vi "Graphene Flexion Test.vi"() -> ()   [LabVIEW 2016]
uses:
  <vilib>/rvi/Emulation/niFpgaGetClockAttributes.vi
  <vilib>/rvi/Emulation/niFpgaSctlEmulationGetInTimedLoop.vi
  <vilib>/rvi/Emulation/niFpgaEmulationReportErrorSimple.vi
  <vilib>/rvi/eio/common/nirviEmuTemplateMethod_errors.vi
  <vilib>/rvi/Emulation/niFpgaCriticalErrorInLSC.vi
  <vilib>/eio/EIONode/EIONode.xnode
  <vilib>/rvi/Analysis/measure/butterworth/XNode/niFpgaButterworthFilter.xnode
panel:
  out "Filtered Signal 1Hz":fxp<+/-,28,9>
  out "Filtered Signal 0.500Hz":fxp<+/-,28,9>
  out "Filtered Signal 0.75Hz":fxp<+/-,28,9>
  out "Unfiltered Signal":sgl
  out "Boolean":bool
  in  "DIO0":bool=TRUE
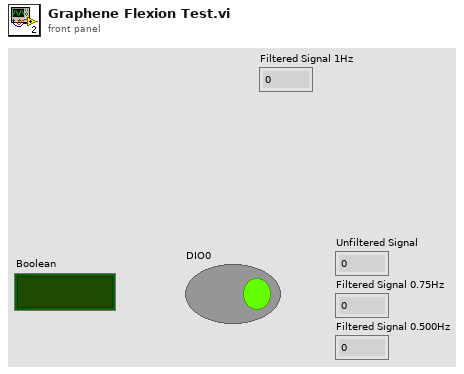
[diagram p1: front panel]
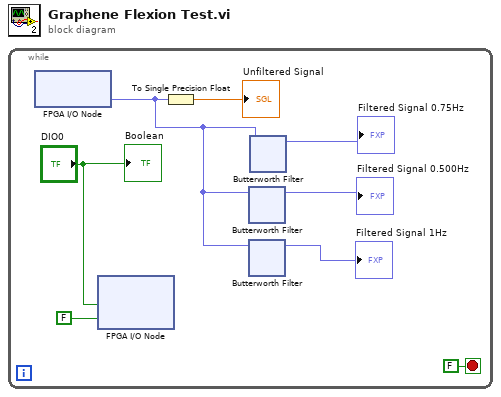
[diagram p0: block diagram]
diagram:
  n1 = while {
    stop <- FALSE ("stop") stop-if-true
    n2 = xnode "FPGA I/O Node"() -> ("AI0"=w2:fxp<+/-,24,5>)  [unwired: 1 in, 1 out]
    n3 = xnode "FPGA I/O Node"("DIO0"="DIO0", "DIO3"=FALSE) -> ()  [unwired: 2 in, 2 out]
    n4 = To Single Precision Float(number=w2) -> (single precision float=→"Unfiltered Signal":sgl)
    n5 = xnode "Butterworth Filter"("input data"=w2) -> ("output data"=→"Filtered Signal 0.500Hz":fxp<+/-,24,5>)  [unwired: 2 in]
    n6 = xnode "Butterworth Filter"("input data"=w2) -> ("output data"=→"Filtered Signal 1Hz":fxp<+/-,24,5>)  [unwired: 2 in]
    n7 = xnode "Butterworth Filter"("input data"=w2) -> ("output data"=→"Filtered Signal 0.75Hz":fxp<+/-,24,5>)  [unwired: 2 in]
    "Boolean" <- "DIO0"
  }
